vi "Button logic.vi"(7 "Enum":enum16{"DI", "AI", "DO", "All", "SG"}(ring)=enum."All", 10 "DAQ ref":T2, 11 "Cluster":T1) -> ()   [LabVIEW 2022 SP3]
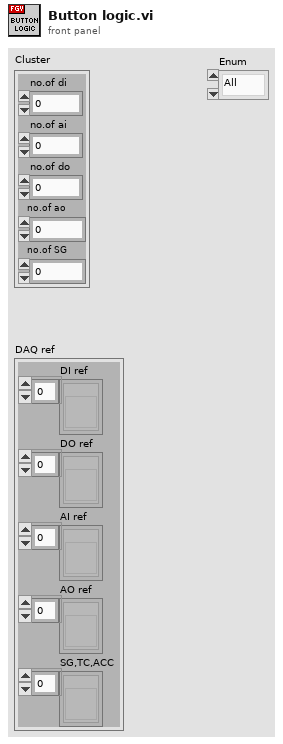
[diagram p1: front panel]
types:
  T1 = cluster{"no.of di":u8, "no.of ai":u8, "no.of do":u8, "no.of ao":u8, "no.of SG":u8}
  T2 = cluster{"DI ref":refnum<vi>[], "DO ref":refnum<vi>[], "AI ref":refnum<vi>[], "AO ref":refnum<vi>[], "SG,TC,ACC":refnum<vi>[]}
  T3 = enum8{"Enabled", "Disabled", "Disabled and Grayed Out"}
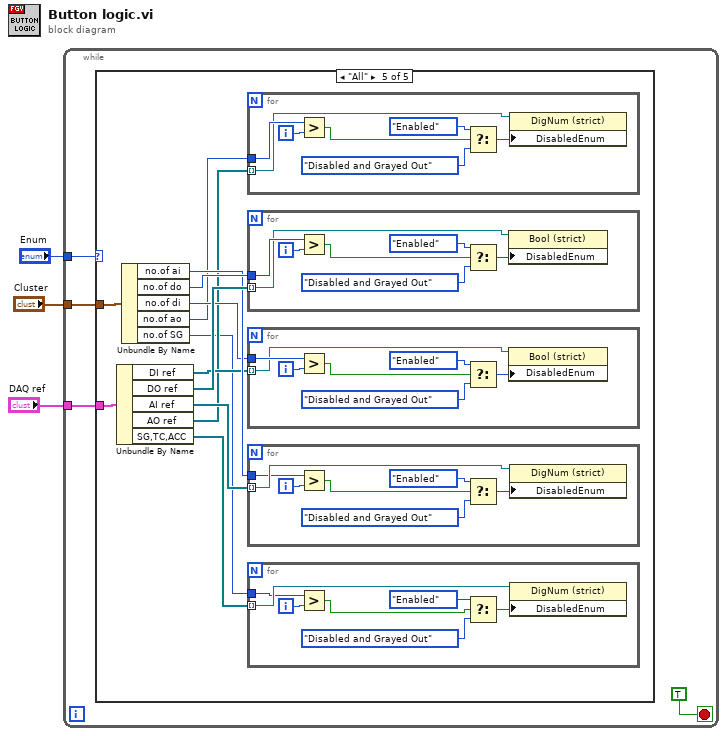
[diagram p0: block diagram]
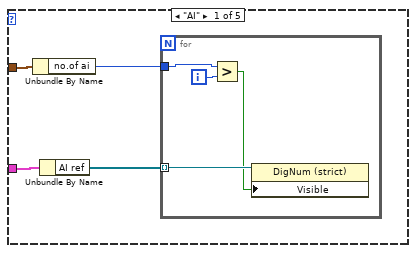
[diagram p2: hidden frame]
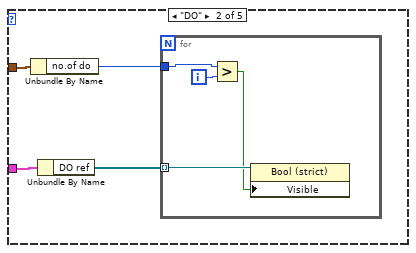
[diagram p3: hidden frame]
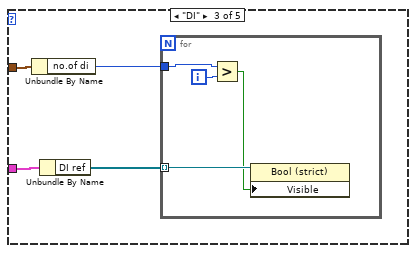
[diagram p4: hidden frame]
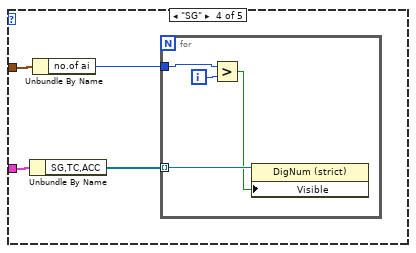
[diagram p5: hidden frame]
diagram:
  n1 = while {
    tunnel: "DAQ ref" -> [w7]
    tunnel: "Enum" -> [w5]
    tunnel: "Cluster" -> [w4]
    stop <- TRUE stop-if-true
    n2 = case shown="\"All\"" w5 {
      tunnel: w7 -> [w11 w19 w27 w32 w51]
      tunnel: w4 -> [w9 w17 w25 w33 w50]
      frame "AI" {
        n3 = Unbundle By Name(w9) -> ("no.of ai"=w8:u8)
        n4 = Unbundle By Name(w11) -> ("AI ref"=w10:refnum<vi>[])
        n5 = for {
          tunnel: w10 -> [w15] mode=indexing
          tunnel: w8 -> [w14]
          i -> [w13]
          n6 = Greater?(x=w14, y=w13) -> (0:w12:bool)
          n7 = property class="DigNum (strict)"(reference=w15, "Visible"=w12) -> ()  [unwired: 1 in, 2 out]
        }
      }
      frame "DO" {
        n8 = Unbundle By Name(w17) -> ("no.of do"=w16:u8)
        n9 = Unbundle By Name(w19) -> ("DO ref"=w18:refnum<vi>[])
        n10 = for {
          tunnel: w18 -> [w23] mode=indexing
          tunnel: w16 -> [w22]
          i -> [w21]
          n11 = Greater?(x=w22, y=w21) -> (0:w20:bool)
          n12 = property class="Bool (strict)"(reference=w23, "Visible"=w20) -> ()  [unwired: 1 in, 2 out]
        }
      }
      frame "DI" {
        n13 = Unbundle By Name(w25) -> ("no.of di"=w24:u8)
        n14 = Unbundle By Name(w27) -> ("DI ref"=w26:refnum<vi>[])
        n15 = for {
          tunnel: w26 -> [w31] mode=indexing
          tunnel: w24 -> [w30]
          i -> [w29]
          n16 = Greater?(x=w30, y=w29) -> (0:w28:bool)
          n17 = property class="Bool (strict)"(reference=w31, "Visible"=w28) -> ()  [unwired: 1 in, 2 out]
        }
      }
      frame "SG" {
        n18 = Unbundle By Name(w32) -> ("SG,TC,ACC"=w35:refnum<vi>[])
        n19 = Unbundle By Name(w33) -> ("no.of ai"=w34:u8)
        n20 = for {
          tunnel: w35 -> [w39] mode=indexing
          tunnel: w34 -> [w38]
          i -> [w37]
          n21 = Greater?(x=w38, y=w37) -> (0:w36:bool)
          n22 = property class="DigNum (strict)"(reference=w39, "Visible"=w36) -> ()  [unwired: 1 in, 2 out]
        }
      }
      frame "All" {
        n23 = Unbundle By Name(w51) -> ("DI ref"=w44:refnum<vi>[], "DO ref"=w48:refnum<vi>[], "AI ref"=w47:refnum<vi>[], "AO ref"=w43:refnum<vi>[], "SG,TC,ACC"=w41:refnum<vi>[])
        n24 = Unbundle By Name(w50) -> ("no.of ai"=w46:u8, "no.of do"=w49:u8, "no.of di"=w45:u8, "no.of ao"=w42:u8, "no.of SG"=w40:u8)
        n25 = for {
          tunnel: w43 -> [w67] mode=indexing
          tunnel: w42 -> [w71]
          i -> [w72]
          n26 = Greater?(x=w71, y=w72) -> (0:w66:bool)
          n27 = Select(t=T3."Enabled" ("Disabled"), s=w66, f=T3."Disabled and Grayed Out" ("Disabled")) -> (s? t:f=w68:T3)
          n28 = property class="DigNum (strict)"(reference=w67, "DisabledEnum"=w68) -> ()  [unwired: 1 in, 2 out]
        }
        n29 = for {
          tunnel: w49 -> [w86]
          tunnel: w48 -> [w84] mode=indexing
          i -> [w85]
          n30 = Greater?(x=w86, y=w85) -> (0:w83:bool)
          n31 = Select(t=T3."Enabled" ("Disabled"), s=w83, f=T3."Disabled and Grayed Out" ("Disabled")) -> (s? t:f=w80:T3)
          n32 = property class="Bool (strict)"(reference=w84, "DisabledEnum"=w80) -> ()  [unwired: 1 in, 2 out]
        }
        n33 = for {
          tunnel: w45 -> [w65]
          tunnel: w44 -> [w63] mode=indexing
          i -> [w64]
          n34 = Greater?(x=w65, y=w64) -> (0:w59:bool)
          n35 = Select(t=T3."Enabled" ("Disabled"), s=w59, f=T3."Disabled and Grayed Out" ("Disabled")) -> (s? t:f=w60:T3)
          n36 = property class="Bool (strict)"(reference=w63, "DisabledEnum"=w60) -> ()  [unwired: 1 in, 2 out]
        }
        n37 = for {
          tunnel: w47 -> [w78] mode=indexing
          tunnel: w46 -> [w77]
          i -> [w79]
          n38 = Greater?(x=w77, y=w79) -> (0:w73:bool)
          n39 = Select(t=T3."Enabled" ("Disabled"), s=w73, f=T3."Disabled and Grayed Out" ("Disabled")) -> (s? t:f=w74:T3)
          n40 = property class="DigNum (strict)"(reference=w78, "DisabledEnum"=w74) -> ()  [unwired: 1 in, 2 out]
        }
        n41 = for {
          tunnel: w41 -> [w57] mode=indexing
          tunnel: w40 -> [w56]
          i -> [w58]
          n42 = Greater?(x=w56, y=w58) -> (0:w52:bool)
          n43 = Select(t=T3."Enabled" ("Disabled"), s=w52, f=T3."Disabled and Grayed Out" ("Disabled")) -> (s? t:f=w53:T3)
          n44 = property class="DigNum (strict)"(reference=w57, "DisabledEnum"=w53) -> ()  [unwired: 1 in, 2 out]
        }
      }
    }
  }
